vi "Robot Systems 2017.vi"(11 "All Robot Commands":T5) -> ()   [LabVIEW 2016]
uses:
  Drive and Climb SS/Drive + Climb Commands 2017.ctl
  Gear Delivery SS/Gear Delivery Commands.ctl
  Conveyor and Shooter SS/Conveyor and Shooter Commands.ctl
  Ball Intake SS/Ball Intake Commands.ctl
  <vilib>/Rock Robotics/WPI/DriverStation/WPI_DriverStationRobotMode2.ctl
  Global Variables/Robot Status.vi
  Robot Global Data.vi
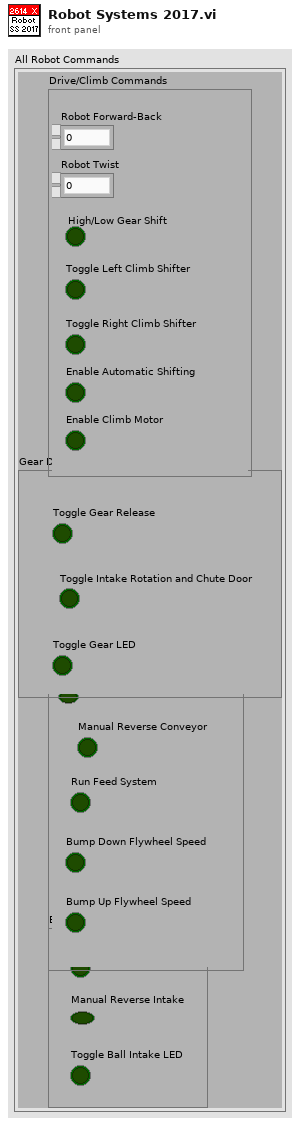
[diagram p1: front panel]
types:
  T1 = typedef "Drive + Climb Commands 2017.ctl" = cluster{"Robot Forward-Back":dbl, "Robot Twist":dbl, "High/Low Gear Shift":bool, "Toggle Left Climb Shifter":bool, "Toggle Right Climb Shifter":bool, "Enable Automatic Shifting":bool, "Enable Climb Motor ":bool}
  T2 = typedef "Gear Delivery Commands.ctl" = cluster{"Toggle Gear Release":bool, "Toggle Intake Rotation and Chute Door":bool, "Toggle Gear LED":bool}
  T3 = typedef "Conveyor and Shooter Commands.ctl" = cluster{"Toggle Shooter":bool, "Manual Reverse Conveyor":bool, "Run Feed System":bool, "Bump Down Flywheel Speed":bool, "Bump Up Flywheel Speed":bool}
  T4 = typedef "Ball Intake Commands.ctl" = cluster{"Toggle Ball Intake":bool, "Manual Reverse Intake":bool, "Toggle Ball Intake LED":bool}
  T5 = cluster{"Drive/Climb Commands":T1, "Gear Delivery Commands":T2, "Shooter and Conveyor Commands":T3, "Ball Intake Commands":T4}
  T6 = typedef "Ball Intake Actuator Out.ctl" = cluster{"Intake Motor Value":dbl}
  T7 = typedef "Conveyor and Shooter Actuator Out.ctl" = cluster{"Conveyor Motor Value":dbl, "Flywheel Motor Value":dbl}
  T8 = typedef "Gear Delivery Actuator Out.ctl" = cluster{"Gear Release":enum16{"Off", "On", "Forward", "Reverse"}, "Gear Intake":enum16{"Off", "On", "Forward", "Reverse"}, "Gear Chute":enum16{"Off", "On", "Forward", "Reverse"}}
  T9 = typedef "Drive Actuator Out 2017.ctl" = cluster{"Left Drive Output":dbl, "Right Drive Output":dbl, "Low/High Gear Shift":enum16{"Off", "On", "Forward", "Reverse"}, "Left Climb Shift":enum16{"Off", "On", "Forward", "Reverse"}, "Right Climb Shift":enum16{"Off", "On", "Forward", "Reverse"}, "Run Climb Motor":dbl}
  T10 = typedef "Conveyor and Shooter Errors.ctl" = errorcluster
  T11 = typedef "Ball Intake Errors.ctl" = errorcluster
  T12 = typedef "Gear Delivery Errors.ctl" = errorcluster
  T13 = typedef "Drive and Climb Errors.ctl" = errorcluster
  T14 = typedef "WPI_DriverStationRobotMode2.ctl" = enum16{"Autonomous Disabled", "Autonomous Enabled", "Teleop Disabled", "Teleop Enabled", "Disconnected", "Finish", "Test Disabled", "Test Enabled", "Emergency Stopped"}
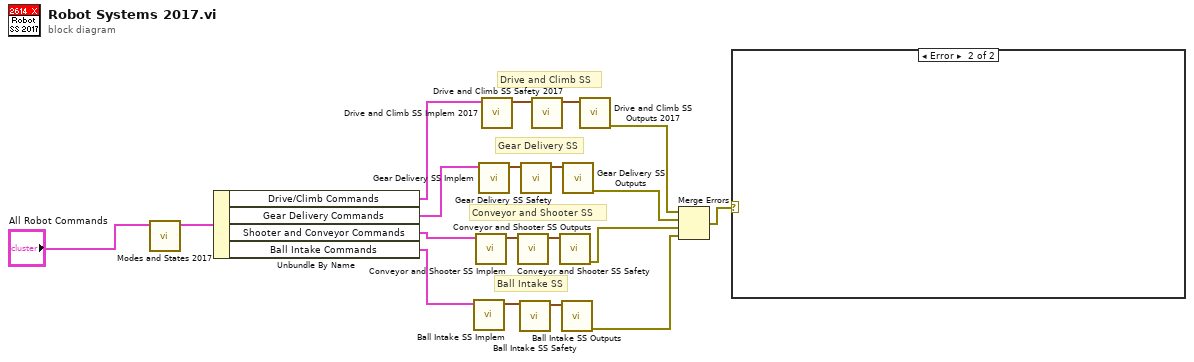
[diagram p0: block diagram]
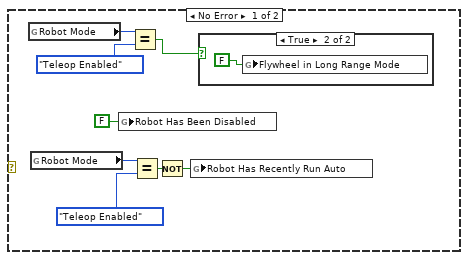
[diagram p2: hidden frame]
diagram:
  # "Gear Delivery SS"
  # "Conveyor and Shooter SS"
  # "Ball Intake SS"
  # "Drive and Climb SS"
  n1 = call "Modes and States 2017.vi"("All Robot Commands In"="All Robot Commands") -> ("All Robot Commands Out"=w12:T5)  [unwired: 10 in]
  n2 = Unbundle By Name(w12) -> ("Drive/Climb Commands"=w11:T1, "Gear Delivery Commands"=w10:T2, "Shooter and Conveyor Commands"=w9:T3, "Ball Intake Commands"=w8:T4)
  n3 = call "Ball Intake SS Implem.vi"("Ball Intake Commands Out"=w8) -> ("Ball Intake Actuator Out"=w17:T6)  [unwired: 10 in]
  n4 = call "Conveyor and Shooter SS Implem.vi"("Shooter and Conveyor Commands In"=w9) -> ("Conveyor and Shooter Actuator Values Out"=w15:T7)  [unwired: 10 in]
  n5 = call "Gear Delivery SS Implem.vi"("Gear Delivery Commands In"=w10) -> ("Gear Delivery Actuators Out"=w7:T8)  [unwired: 10 in]
  n6 = call "Drive and Climb SS Implem 2017.vi"("Robot Commands"=w11) -> ("Drive Actuator Out"=w19:T9)  [unwired: 10 in]
  n7 = call "Conveyor and Shooter SS Safety.vi"("Conveyor and Shooter Actuator Values In"=w15) -> ("Conveyor and Shooter Actuator Values Out"=w14:T7)  [unwired: 10 in]
  n8 = call "Ball Intake SS Safety.vi"("Ball Intake Actuator In"=w17) -> ("Ball Intake Actuator Out"=w16:T6)  [unwired: 10 in]
  n9 = call "Gear Delivery SS Safety.vi"("Gear Delivery Actuator In"=w7) -> ("Gear Delivery Actuator Out"=w6:T8)  [unwired: 10 in]
  n10 = call "Drive and Climb SS Safety 2017.vi"("Drive Actuator In"=w19) -> ("Drive Actuator Out"=w18:T9)  [unwired: 10 in]
  n11 = call "Conveyor and Shooter SS Outputs.vi"("Conveyor and Shooter Actuator Values In"=w14) -> ("error out"=w4:T10)  [unwired: 10 in]
  n12 = call "Ball Intake SS Outputs.vi"("Ball Intake Actuator In"=w16) -> ("error out"=w5:T11)  [unwired: 10 in]
  n13 = call "Gear Delivery SS Outputs.vi"("Gear Delivery Actuator In"=w6) -> ("error out"=w3:T12)  [unwired: 10 in]
  n14 = call "Drive and Climb SS Outputs 2017.vi"("Drive Actuator In"=w18) -> ("error out"=w2:T13)  [unwired: 10 in]
  n15 = Merge Errors(w2, w3, w4, w5) -> (w1:errorcluster)
  n16 = case shown="Error" w1 {
    frame No Error {
      n17 = global read "Robot Global Data.vi" "Robot Mode"() -> (w22:T14)
      n18 = global read "Robot Global Data.vi" "Robot Mode"() -> (w26:T14)
      n19 = global write "Robot Status.vi" "Robot Has Been Disabled"(FALSE ("Robot Has Been Disabled")) -> ()
      n20 = Equal?(x=w22, y=WPI_DriverStationRobotMode2."Teleop Enabled") -> (x = y?=w20:bool)
      n21 = Equal?(x=w26, y=WPI_DriverStationRobotMode2."Teleop Enabled") -> (x = y?=w24:bool)
      n22 = Not(x=w24) -> (.not. x?=w23:bool)
      n23 = global write "Robot Status.vi" "Robot Has Recently Run Auto"(w23) -> ()
      n24 = case shown="True" w20 {
        frame False {
        }
        frame True {
          n25 = global write "Robot Status.vi" "Flywheel in Long Range Mode"(FALSE) -> ()
        }
      }
    }
    frame Error {
    }
  }
